vi "IQBurst_memo_Create.vi"(8 "error in (no error)":errorcluster, 10 "burst name":string, 11 "reference in":refnum<class "IQBurst_memo.lvclass">) -> (0 "error out":errorcluster, 3 "reference out":refnum<class "IQBurst_memo.lvclass">)   [LabVIEW 2019, in "IQBurst_memo.lvclass"]
doc: "Constructor."
uses:
  IQBurst_memo.lvclass
  C:/Program Files/National Instruments/LabVIEW 2019/vi.lib/addons/_AddQ/G#Object/G#Object.lvclass
  C:/Barkhausen mmWave radar/Development/LV/Barkhausen mmWave hardware control/Host/SubVIs/mmWave data_class/mmWave data.lvclass
  <vilib>/Utility/error.llb/Error Cluster From Error Code.vi
  <vilib>/ErrorRing/Error Ring.xnode
  <vilib>/addons/_AddQ/G#Object/G#Object.lvclass
  mmWave data_class/mmWave data.lvclass
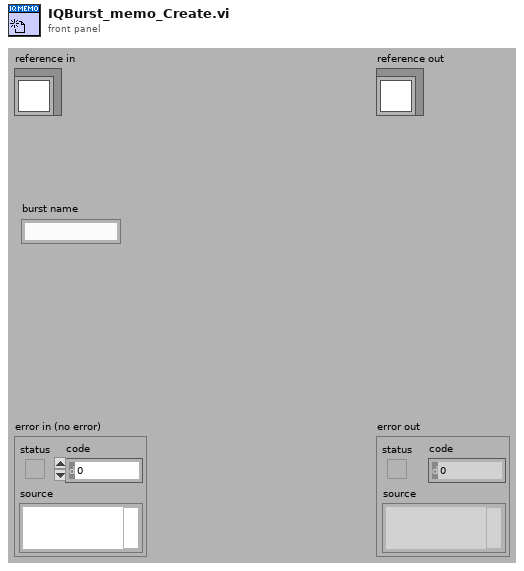
[diagram p1: front panel]
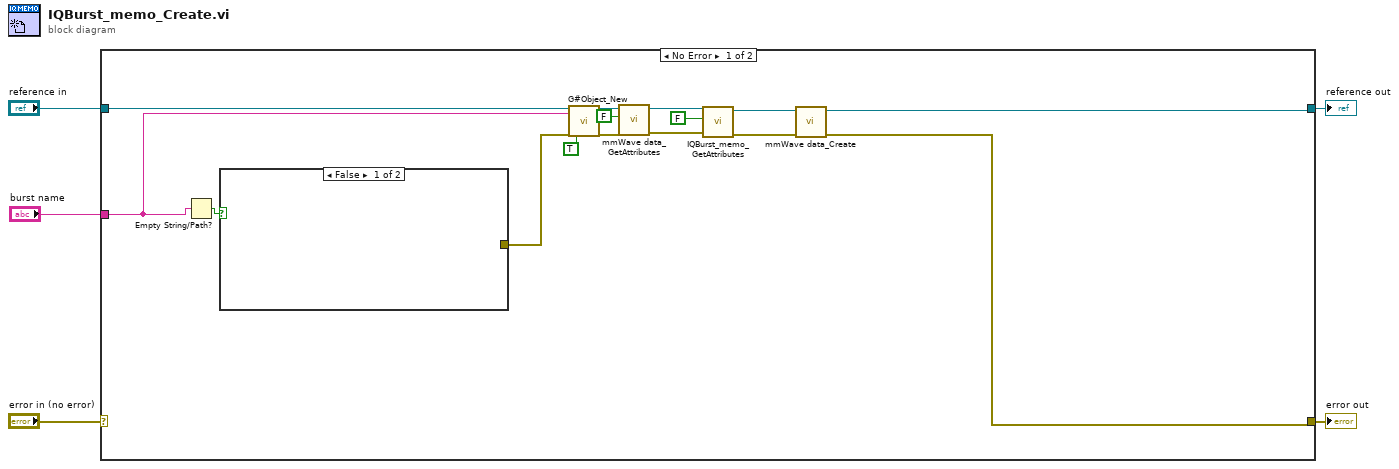
[diagram p0: block diagram]
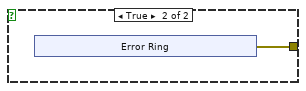
[diagram p2: hidden frame]
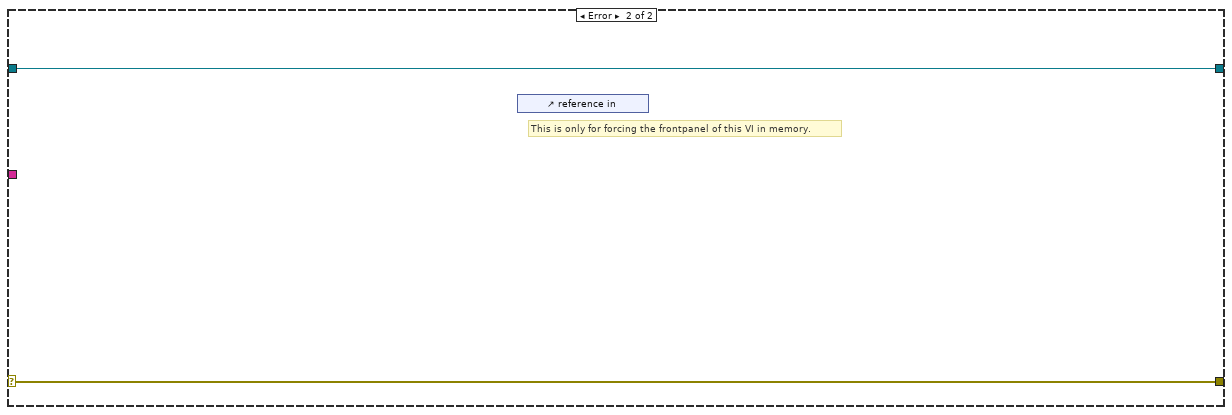
[diagram p3: hidden frame]
diagram:
  n1 = case shown="No Error" "error in (no error)" {
    selector: "error in (no error)" -> [_ w28]
    tunnel: [w13 w28] -> w4
    tunnel: [w14 w27] -> w2
    tunnel: "reference in" -> [w20 w27]
    tunnel: "burst name" -> [w8 _]
    frame No Error {
      n2 = Empty String/Path?(string/path=w8) -> (empty?=w7:bool)
      n3 = case shown="False" w7 {
        tunnel: [_ w21] -> w6
        frame False {
        }
        frame True {
          n4 = xnode "Error Ring"() -> ("error out"=w21:errorcluster)
        }
      }
      n5 = call <vilib>:"G#Object_New.vi"("reference in"=w20, "object name"=w8, "error in (no error)"=w6, "user counter (T)?"=TRUE ("User Counter")) -> ("reference out"=w16:refnum<class "IQBurst_memo.lvclass">, "error out"=w10:errorcluster)  [unwired: 13 in, 1 out]
      n6 = call "mmWave data_GetAttributes.vi"("error in (no error)"=w10, "return data? (T)"=FALSE, "reference in"=w16) -> ("error out"=w9:errorcluster, "reference out"=w12:refnum<class "IQBurst_memo.lvclass">)  [unwired: 5 in, 2 out]
      n7 = call "IQBurst_memo_GetAttributes.vi"("error in (no error)"=w9, "return data? (T)"=FALSE ("return data"), "reference in"=w12) -> ("error out"=w18:errorcluster, "reference out"=w15:refnum<class "IQBurst_memo.lvclass">)  [unwired: 5 in, 2 out]
      n8 = call "mmWave data_Create.vi"("error in (no error)"=w18, "reference in"=w15) -> ("error out"=w13:errorcluster, "reference out"=w14:refnum<class "IQBurst_memo.lvclass">)  [unwired: 8 in]
    }
    frame Error {
      # "This is only for forcing the frontpanel of this VI in memory."
      n9 = control-ref of="reference in"() -> ()  [unwired: 1 out]
    }
  }
  "error out" <- w4
  "reference out" <- w2
